vi "ConvertBarWidthsToBars.vi"(8 "error in (no error)":errorcluster, 10 "BarWidths":u8[][](array[numeric]), 11 "BarCode in":refnum<class "BarCode.lvclass">) -> (0 "error out":errorcluster, 2 "Bars":T1[][](array[typedef]), 3 "BarCode out":refnum<class "BarCode.lvclass">)   [LabVIEW 2013, in "BarCodes.lvlib" / "BarCode.lvclass"]
uses:
  BarCode.lvclass
  Bar.ctl
  Read Dark Color.vi
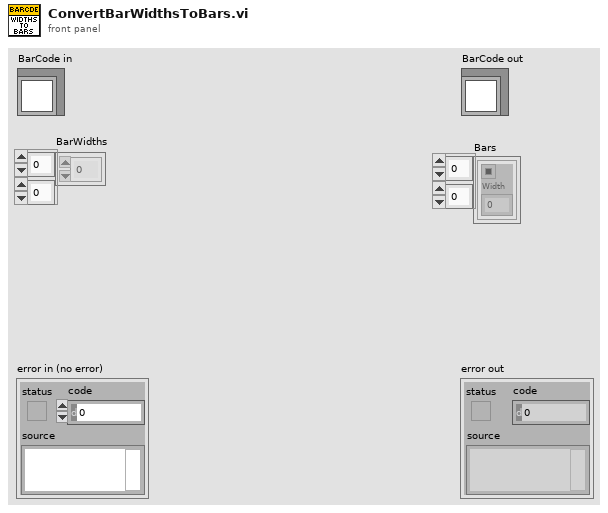
[diagram p1: front panel]
types:
  T1 = typedef "BarCodes.lvlib/BarCode.lvclass/Bar.ctl" = cluster{"Color":u32, "Width":u8}
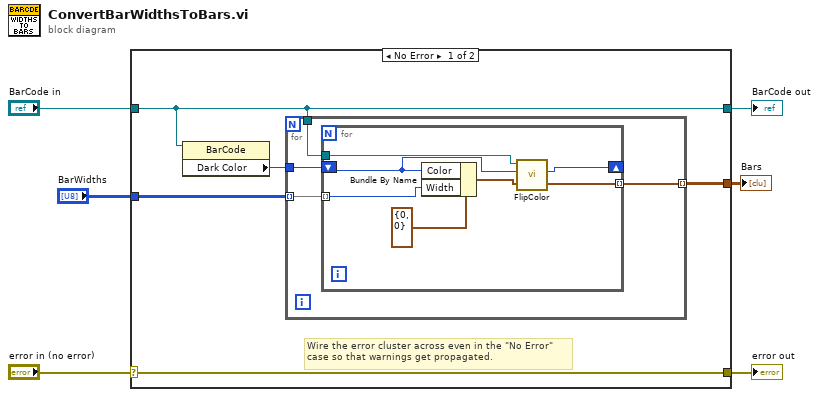
[diagram p0: block diagram]
diagram:
  n1 = case shown="No Error" "error in (no error)" {
    selector: "error in (no error)" -> [w11 w23]
    tunnel: [w11 w23] -> w5
    tunnel: [w9 w22] -> w3
    tunnel: "BarCode in" -> [w9 w22]
    tunnel: "BarWidths" -> [w10 _]
    tunnel: [w7 _] -> w1
    frame No Error {
      # "Wire the error cluster across even in the \"No Error\"\ncase so that warnings get propagated."
      n2 = property class="BarCode"(reference=w9) -> ("Dark Color"=w8:u32)  [unwired: 1 in, 2 out]
      n3 = for {
        tunnel: w9 -> [w15]
        tunnel: w10 -> [w13] mode=indexing
        tunnel: w8 -> [w14]
        tunnel: [w12] -> w7 mode=indexing
        n4 = for {
          tunnel: w15 -> [w20]
          tunnel: w13 -> [w17] mode=indexing
          shift-right: [w18] -> _
          shift-left: w14 -> [w19]
          tunnel: [w16] -> w12 mode=indexing
          n5 = Bundle By Name(cluster=T1 {"Color"=0, "Width"=0} ("Bar"), "Color"=w19, "Width"=w17) -> (w16:T1)
          n6 = call-dynamic "FlipColor.vi"("Current Color"=w19, "BarCode in"=w20) -> ("Next color"=w18:u32)  [unwired: 8 in, 1 out]
        }
      }
    }
    frame Error {
    }
  }
  "error out" <- w5
  "BarCode out" <- w3
  "Bars" <- w1
